vi "Write Prompt UI VI Ref.vi"(8 "error in (no error)":errorcluster, 10 "Prompt UI VI Ref":refnum<vi>, 11 "Abstract Sensor in":refnum<class "Abstract Sensor.lvclass">) -> (0 "error out":errorcluster, 3 "Abstract Sensor out":refnum<class "Abstract Sensor.lvclass">)   [LabVIEW 2014]
uses:
  Abstract Sensor.lvclass
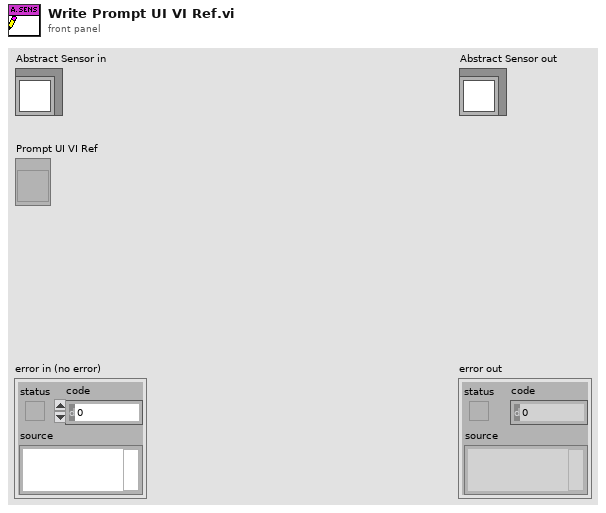
[diagram p1: front panel]
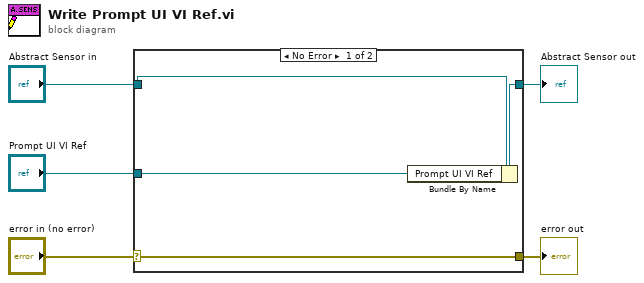
[diagram p0: block diagram]
diagram:
  n1 = case shown="No Error" "error in (no error)" {
    selector: "error in (no error)" -> [w9 w10]
    tunnel: [w9 w10] -> w4
    tunnel: [w7 w11] -> w2
    tunnel: "Abstract Sensor in" -> [w8 w11]
    tunnel: "Prompt UI VI Ref" -> [w6 _]
    frame No Error {
      n2 = Bundle By Name(cluster=w8, "Prompt UI VI Ref"=w6) -> (w7:refnum<class "Abstract Sensor.lvclass">)
    }
    frame Error {
    }
  }
  "error out" <- w4
  "Abstract Sensor out" <- w2
